vi "U32 1D to Data Type.vi"(8 "error in (no error)":errorcluster, 11 "U32 1D":u32[](array[numeric])) -> (0 "error out":errorcluster, 3 "Boolean out":refnum<class "U32 1D.lvclass">)   [LabVIEW 2019, in "U32 1D.lvclass"]
uses:
  <vilib>/gpm_packages/@cs/data-type-serializer/source/U32 1D/U32 1D.lvclass
  <vilib>/gpm_packages/@cs/data-type-serializer/source/U32 1D/U32 1D.lvclass/U32 1D.ctl
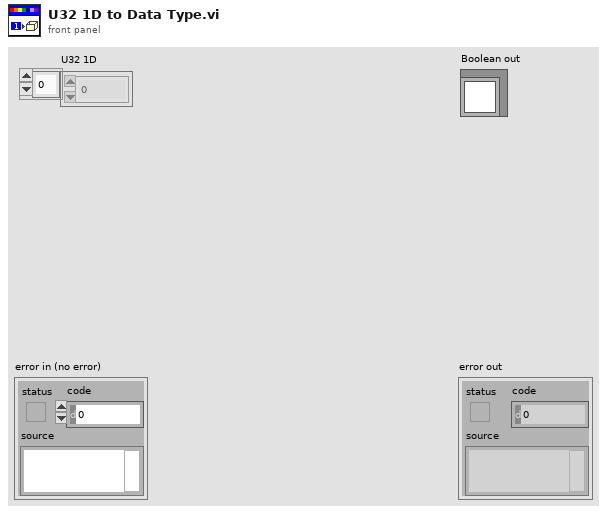
[diagram p1: front panel]
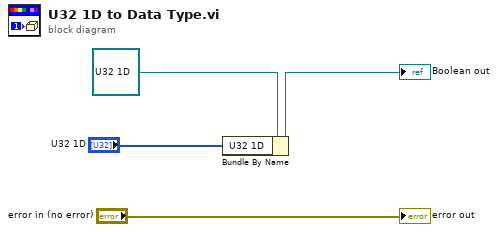
[diagram p0: block diagram]
diagram:
  n1 = Bundle By Name(cluster=refnum<class "U32 1D.lvclass"> refnum ("Boolean in"), "U32 1D"="U32 1D") -> (→"Boolean out":refnum<class "U32 1D.lvclass">)
  "error out" <- "error in (no error)"
